vi "PH_Beckhoff_StepMot.destructor.vi"(0 "i ref in":refnum<vi>, 5 "error in(no error)":errorcluster) -> (19 "error out":errorcluster)   [LabVIEW 2014, in "PH_Beckhoff_StepMot.lvlib"]
doc: "This is the destructor of a class.\n\nLicense Agreement for this software:\n\nCopyright (C)\nGesellschaft für Schwerionenforschung, GSI\nPlanckstr. 1\n64291 Darmstadt\nGermany\n\nContact: D.Beck@gsi.de \n\nThis program is free software; you can redistribute it and/or modify it under the terms of the \nGNU General Public License as published by the Free Software Foundation; either version 2 of \nthe license, or (at your option) any later version.\n\nThis program is distributed in the hope that it will be useful, but WITHOUT ANY WARRANTY; \nwithout even the implied warranty of MERCHANTABILITY or FITNESS FOR A PARTICULAR PURPOSE. See the GNU General License for more details (http://www.gnu.org).\n\nGesellschaft für Schwerionenforschung, GSI\nPlanckstr. 1, 64291 Darmstadt, Germany\nFor all questions and ideas contact: M.Richter@gsi.de, H.Brand@gsi.de or D.Beck@gsi.de.\nLast update: 16-JUN-2004"
uses:
  PH_Beckhoff_StepMot.lvlib
  PH_Beckhoff/PH_Beckhoff.lvlib
  PH_Basics/PH_Stepmotor_BaseClass/PH_Stepmotor_BaseClass.lvlib
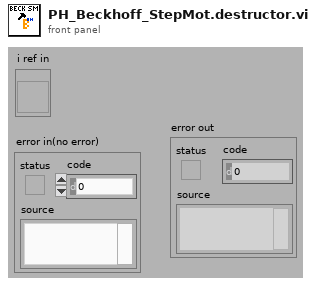
[diagram p1: front panel]
types:
  T1 = enum16{"SetAttribute", "GetAttribute", "CreateAttribute", "DestroyAttribute", "DestroyAllAtributes"}
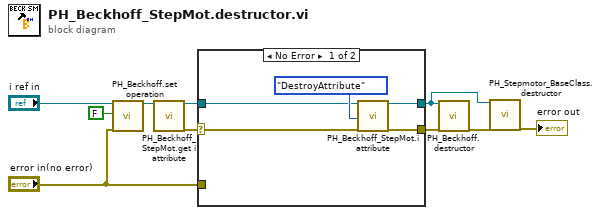
[diagram p0: block diagram]
diagram:
  n1 = call "PH_Beckhoff.set operation.vi"("VI in"="i ref in", "operation?"=FALSE, "error in (no error)"="error in(no error)") -> ("VI out"=w2:refnum<vi>)  [unwired: 15 in, 1 out]
  n2 = call "PH_Beckhoff_StepMot.get i attribute.vi"("i ref in"=w2) -> ("i ref out"=w8:refnum<vi>, "error out"=w7:errorcluster)  [unwired: 16 in, 1 out]
  n3 = case shown="No Error" w7 {
    selector: w7 -> [w11 _]
    tunnel: [w14 w17] -> w6
    tunnel: [w13 w16] -> w9
    tunnel: w8 -> [w12 w17]
    tunnel: "error in(no error)" -> [_ w16]
    frame No Error {
      n4 = call "PH_Beckhoff_StepMot.i attribute.vi"("VI Refnum"=w12, "Action"=T1."DestroyAttribute", "error in (no error)"=w11) -> ("VI Refnum out"=w14:refnum<vi>, "error out"=w13:errorcluster)  [unwired: 14 in, 1 out]
    }
    frame Error {
    }
  }
  n5 = call "PH_Beckhoff.destructor.vi"("i ref in"=w6, "error in(no error)"=w9) -> ("error out"=w10:errorcluster)  [unwired: 17 in]
  n6 = call "PH_Stepmotor_BaseClass.destructor.vi"("i ref in"=w6, "error in"=w10) -> ("error out"=→"error out":errorcluster)  [unwired: 17 in]
